vi "ChangeTCSServer.vi"() -> (0 "error out":errorcluster)   [LabVIEW 2015]
uses:
  Utils/ChangeTCS.ctl
  Users/Sherman/Desktop/BETA_GSCS/Systems/SystemUtil/Command.ctl
  TCPServer/TCP_Global.vi
panel:
  in  "Last Command":string
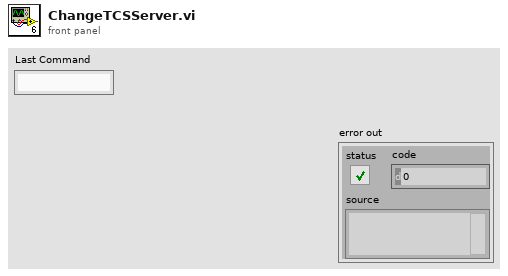
[diagram p1: front panel]
types:
  T1 = typedef "ChangeTCS.ctl" = cluster{"Command":string, "TCS":cluster{"Comp Mirror":bool, "RA":string, "DEC":string, "Epoch":string}}
  T2 = typedef "Command.ctl" = cluster{"Command":string, "Parameter":string}
  T3 = cluster{"Comp Mirror":bool, "RA":string, "DEC":string, "Epoch":string}
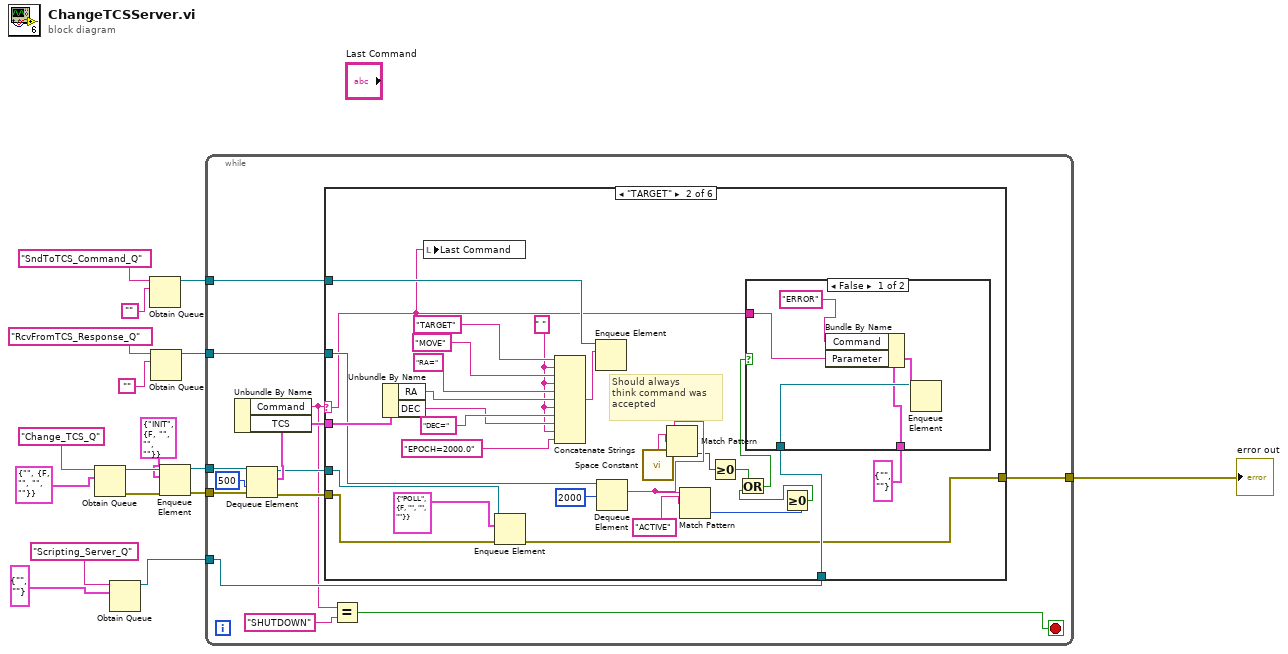
[diagram p0: block diagram]
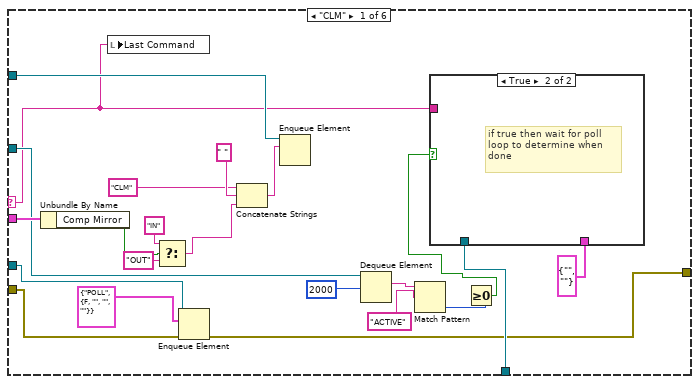
[diagram p2: hidden frame]
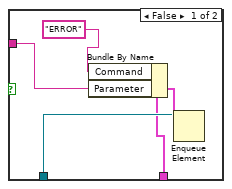
[diagram p3: hidden frame]
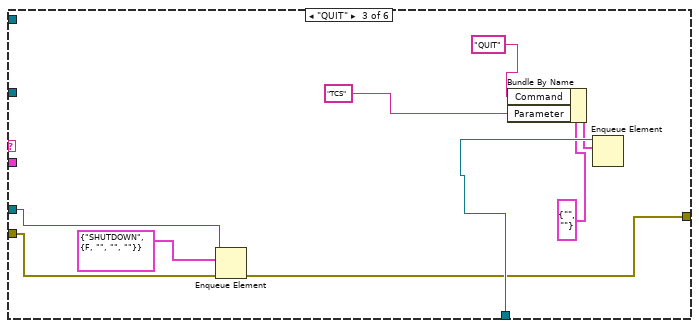
[diagram p5: hidden frame]
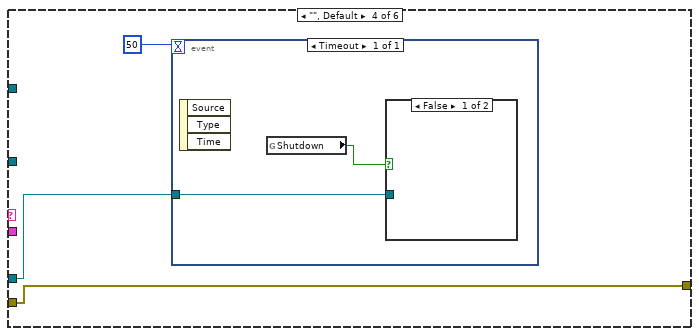
[diagram p6: hidden frame]
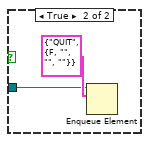
[diagram p7: hidden frame]
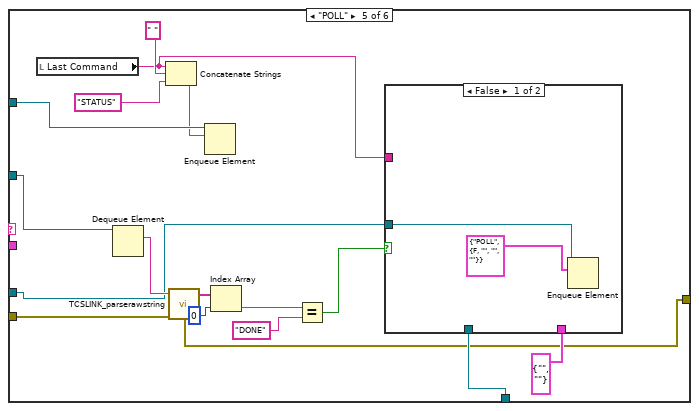
[diagram p8: hidden frame]
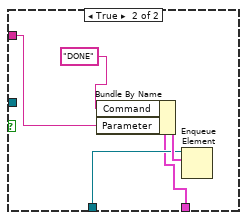
[diagram p9: hidden frame]
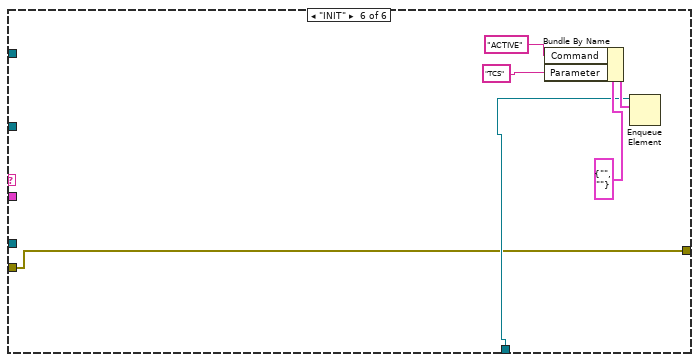
[diagram p10: hidden frame]
diagram:
  n1 = Obtain Queue(name (unnamed)="Change_TCS_Q", element data type=T1 {"Command"="", "TCS"={"Comp Mirror"=FALSE, "RA"="", "DEC"="", "Epoch"=""}} ("Cluster")) -> (queue out=w15:refnum<queue>, error out=w14:errorcluster)  [unwired: 3 in, 1 out]
  n2 = Obtain Queue(name (unnamed)="Scripting_Server_Q", element data type=T2 {"Command"="", "Parameter"=""} ("Command")) -> (queue out=w3:refnum<queue>)  [unwired: 3 in, 2 out]
  n3 = Obtain Queue(name (unnamed)="SndToTCS_Command_Q", element data type="") -> (queue out=w7:refnum<queue>)  [unwired: 3 in, 2 out]
  n4 = Obtain Queue(name (unnamed)="RcvFromTCS_Response_Q", element data type="") -> (queue out=w6:refnum<queue>)  [unwired: 3 in, 2 out]
  n5 = Enqueue Element(queue=w15, element=T1 {"Command"="INIT", "TCS"={"Comp Mirror"=FALSE, "RA"="", "DEC"="", "Epoch"=""}} ("Cluster"), error in (no error)=w14) -> (queue out=w13:refnum<queue>, error out=w12:errorcluster)  [unwired: 1 in, 1 out]
  n6 = while {
    tunnel: w13 -> [w31]
    tunnel: w12 -> [w30]
    tunnel: w7 -> [w27]
    tunnel: w6 -> [w26]
    tunnel: w3 -> [w24]
    tunnel: [w18] -> w1
    stop <- w19 stop-if-true
    n7 = Dequeue Element(queue=w31, timeout in ms (-1)=500, error in (no error)=w30) -> (queue out=w23:refnum<queue>, element=w29:T1, error out=w25:errorcluster)  [unwired: 1 out]
    n8 = Unbundle By Name(w29) -> ("Command"=w20:string, "TCS"=w28:T3)
    n9 = case shown="\"TARGET\"" w20 {
      selector: w20 -> [w38 w74 _ _ _ _]
      tunnel: w28 -> [w51 w85 _ _ _ _]
      tunnel: w27 -> [w46 w81 _ _ w123 _]
      tunnel: w26 -> [w44 w79 _ _ w119 _]
      tunnel: w25 -> [w40 w76 w98 w103 w108 w131]
      tunnel: w24 -> [w42 w78 w100 _ w111 w132]
      tunnel: w23 -> [w37 w73 w96 w101 w112 _]
      tunnel: [w36 w65 w92 w103 w108 w131] -> w18
      frame "CLM" {
        n10 = Unbundle By Name(w51) -> ("Comp Mirror"=w35:bool)
        n11 = local write "Last Command"(w38) -> ()
        n12 = Select(t="IN", s=w35, f="OUT") -> (s? t:f=w32:string)
        n13 = Enqueue Element(queue=w37, element=T1 {"Command"="POLL", "TCS"={"Comp Mirror"=FALSE, "RA"="", "DEC"="", "Epoch"=""}} ("Cluster"), error in (no error)=w40) -> (error out=w36:errorcluster)  [unwired: 1 in, 2 out]
        n14 = Concatenate Strings("CLM", " " ("string"), w32) -> (w45:string)
        n15 = Enqueue Element(queue=w46, element=w45) -> ()  [unwired: 2 in, 3 out]
        n16 = Dequeue Element(queue=w44, timeout in ms (-1)=2000) -> (element=w50:string)  [unwired: 1 in, 3 out]
        n17 = Match Pattern(string=w50, regular expression="ACTIVE") -> (offset past match=w47:i32)  [unwired: 1 in, 3 out]
        n18 = Greater Or Equal To 0?(x=w47) -> (x >= 0?=w43:bool)
        n19 = case shown="True" w43 {
          tunnel: w42 -> [w56 _]
          tunnel: w38 -> [w55 _]
          tunnel: T2 {"Command"="", "Parameter"=""} ("Command") -> [w54 _]
          frame False {
            n20 = Bundle By Name(cluster=w54, "Command"="ERROR", "Parameter"=w55) -> (w58:T2)
            n21 = Enqueue Element(queue=w56, element=w58) -> ()  [unwired: 2 in, 3 out]
          }
          frame True {
            # "if true then wait for poll\nloop to determine when\ndone"
          }
        }
      }
      frame "TARGET" {
        w67 = " " ("string")
        # "Should always \nthink command was\naccepted"
        n22 = Unbundle By Name(w85) -> ("RA"=w70:string, "DEC"=w68:string)
        n23 = local write "Last Command"(w74) -> ()
        n24 = Enqueue Element(queue=w73, element=T1 {"Command"="POLL", "TCS"={"Comp Mirror"=FALSE, "RA"="", "DEC"="", "Epoch"=""}} ("Cluster"), error in (no error)=w76) -> (error out=w65:errorcluster)  [unwired: 1 in, 2 out]
        n25 = Concatenate Strings("TARGET", w67, "MOVE", w67, "RA=", w70, w67, "DEC=", w68, w67, "EPOCH=2000.0") -> (w80:string)
        n26 = Enqueue Element(queue=w81, element=w80) -> ()  [unwired: 2 in, 3 out]
        n27 = Dequeue Element(queue=w79, timeout in ms (-1)=2000) -> (element=w63:string)  [unwired: 1 in, 3 out]
        n28 = call <vilib>:"Space Constant.vi"() -> ("String"=w64:string)
        n29 = Match Pattern(string=w63, regular expression=w64) -> (offset past match=w62:i32)  [unwired: 1 in, 3 out]
        n30 = Match Pattern(string=w63, regular expression="ACTIVE") -> (offset past match=w82:i32)  [unwired: 1 in, 3 out]
        n31 = Greater Or Equal To 0?(x=w62) -> (x >= 0?=w61:bool)
        n32 = Greater Or Equal To 0?(x=w82) -> (x >= 0?=w59:bool)
        n33 = Or(x=w61, y=w59) -> (x .or. y?=w60:bool)
        n34 = case shown="False" w60 {
          tunnel: w78 -> [w89 _]
          tunnel: w74 -> [w88 _]
          tunnel: T2 {"Command"="", "Parameter"=""} ("Command") -> [w87 _]
          frame False {
            n35 = Bundle By Name(cluster=w87, "Command"="ERROR", "Parameter"=w88) -> (w91:T2)
            n36 = Enqueue Element(queue=w89, element=w91) -> ()  [unwired: 2 in, 3 out]
          }
          frame True {
            # "if true wait for poll loop\nto find out when move is done"
          }
        }
      }
      frame "QUIT" {
        n37 = Enqueue Element(queue=w96, element=T1 {"Command"="SHUTDOWN", "TCS"={"Comp Mirror"=FALSE, "RA"="", "DEC"="", "Epoch"=""}} ("Cluster"), error in (no error)=w98) -> (error out=w92:errorcluster)  [unwired: 1 in, 2 out]
        n38 = Bundle By Name(cluster=T2 {"Command"="", "Parameter"=""} ("Command"), "Command"="QUIT", "Parameter"="TCS") -> (w94:T2)
        n39 = Enqueue Element(queue=w100, element=w94) -> ()  [unwired: 2 in, 3 out]
      }
      frame "", Default {
        n40 = event shown="[0] Timeout" {
          selector: _ -> [_]
          dyn-events: _ -> [_]
          timeout: 50 -> [_]
          tunnel: w101 -> [w105]
          event Timeout {
            n41 = event-data() -> ()  [unwired: 1 in, 3 out]
            n42 = global read "TCP_Global.vi" "Shutdown"() -> (w104:bool)
            n43 = case shown="False" w104 {
              tunnel: w105 -> [_ w106]
              frame False {
              }
              frame True {
                n44 = Enqueue Element(queue=w106, element=T1 {"Command"="QUIT", "TCS"={"Comp Mirror"=FALSE, "RA"="", "DEC"="", "Epoch"=""}} ("Cluster")) -> ()  [unwired: 2 in, 3 out]
              }
            }
          }
        }
      }
      frame "POLL" {
        n45 = local read "Last Command"() -> (w110:string)
        n46 = Dequeue Element(queue=w119) -> (element=w118:string)  [unwired: 2 in, 3 out]
        n47 = Concatenate Strings(w110, " " ("string"), "STATUS") -> (w120:string)
        n48 = call "TCSLINK_parserawstring.vi"("Raw String"=w118) -> ("Array"=w117:string[])  [unwired: 4 in]
        n49 = Enqueue Element(queue=w123, element=w120) -> ()  [unwired: 2 in, 3 out]
        n50 = Index Array(array=w117, index=0) -> (element=w115:string)
        n51 = Equal?(x=w115, y="DONE") -> (x = y?=w113:bool)
        n52 = case shown="False" w113 {
          tunnel: w112 -> [w124 _]
          tunnel: w111 -> [_ w127]
          tunnel: w110 -> [_ w128]
          tunnel: T2 {"Command"="", "Parameter"=""} ("Command") -> [_ w126]
          frame False {
            n53 = Enqueue Element(queue=w124, element=T1 {"Command"="POLL", "TCS"={"Comp Mirror"=FALSE, "RA"="", "DEC"="", "Epoch"=""}} ("Cluster")) -> ()  [unwired: 2 in, 3 out]
          }
          frame True {
            n54 = Bundle By Name(cluster=w126, "Command"="DONE", "Parameter"=w128) -> (w129:T2)
            n55 = Enqueue Element(queue=w127, element=w129) -> ()  [unwired: 2 in, 3 out]
          }
        }
      }
      frame "INIT" {
        n56 = Bundle By Name(cluster=T2 {"Command"="", "Parameter"=""} ("Command"), "Command"="ACTIVE", "Parameter"="TCS") -> (w134:T2)
        n57 = Enqueue Element(queue=w132, element=w134) -> ()  [unwired: 2 in, 3 out]
      }
    }
    n58 = Equal?(x=w20, y="SHUTDOWN") -> (x = y?=w19:bool)
  }
  "error out" <- w1
